vi "Get Enqueuer by TabName.vi"(10 "Page":string, 11 "ActorMeter":refnum<class "ActorMeter.lvclass">) -> (3 "Enqueuer":refnum<class "Message Enqueuer.lvclass">)   [LabVIEW 2014]
uses:
  ActorMeter.lvclass
  <vilib>/ActorFramework/Message Enqueuer/Message Enqueuer.lvclass
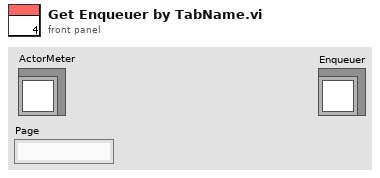
[diagram p1: front panel]
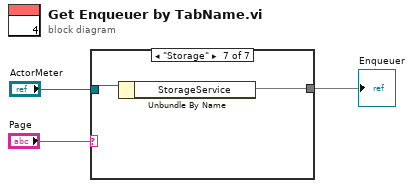
[diagram p0: block diagram]
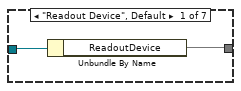
[diagram p2: hidden frame]
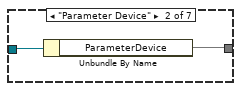
[diagram p3: hidden frame]
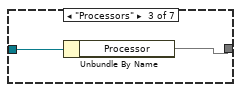
[diagram p4: hidden frame]
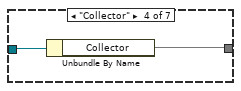
[diagram p5: hidden frame]
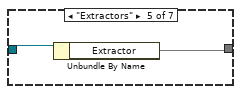
[diagram p6: hidden frame]
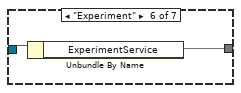
[diagram p7: hidden frame]
diagram:
  n1 = case shown="\"Storage\"" "Page" {
    tunnel: "ActorMeter" -> [w5 w6 w8 w11 w13 w15 w17]
    tunnel: [w4 w7 w9 w10 w12 w14 w16] -> w1
    frame "Readout Device", Default {
      n2 = Unbundle By Name(w5) -> ("ReadoutDevice"=w4)
    }
    frame "Parameter Device" {
      n3 = Unbundle By Name(w6) -> ("ParameterDevice"=w7)
    }
    frame "Processors" {
      n4 = Unbundle By Name(w8) -> ("Processor"=w9)
    }
    frame "Collector" {
      n5 = Unbundle By Name(w11) -> ("Collector"=w10)
    }
    frame "Extractors" {
      n6 = Unbundle By Name(w13) -> ("Extractor"=w12)
    }
    frame "Experiment" {
      n7 = Unbundle By Name(w15) -> ("ExperimentService"=w14)
    }
    frame "Storage" {
      n8 = Unbundle By Name(w17) -> ("StorageService"=w16)
    }
  }
  "Enqueuer" <- w1
